vi "Pick Up and Go.vi"(0 "Feet":dbl=10.0 format="%#_13g") -> ()   [LabVIEW 2014]
panel:
  in  "Time":i32
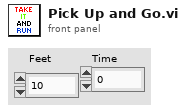
[diagram p1: front panel]
types:
  T1 = enum16{"Move Forward", "Move Backward", "Strafe Right", "Strafe Left"}
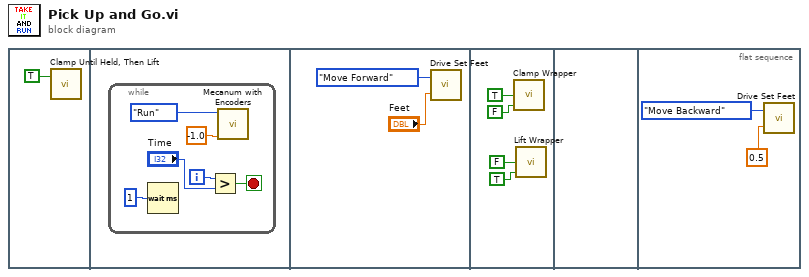
[diagram p0: block diagram]
diagram:
  n1 = flat-sequence {
    frame #0 {
      n2 = call "Clamp Until Held, Then Lift.vi"("Clamp + Lift"=TRUE) -> ()  [unwired: 2 in]
    }
    frame #1 {
      n3 = while {
        i -> [w4]
        stop <- w6 stop-if-true
        n4 = Wait (ms)(milliseconds to wait=u32 1) -> ()  [unwired: 1 out]
        n5 = Greater?(x=w4, y="Time") -> (0:w6:bool)
        n6 = call "Mecanum with Encoders.vi"("Turn"=-1.0, "Mode"=enum8{"Start", "Run", "Finish"}."Run") -> ()  [unwired: 8 in, 1 out]
      }
    }
    frame #2 {
      n7 = call "Drive Set Feet.vi"("Feet"="Feet", "Direction"=T1."Move Forward") -> ()  [unwired: 1 out]
    }
    frame #3 {
      n8 = call "Clamp Wrapper.vi"("In"=FALSE, "Out"=TRUE) -> ()  [unwired: 1 in]
      n9 = call "Lift Wrapper.vi"("Down"=TRUE, "Up"=FALSE) -> ()  [unwired: 1 in]
    }
    frame #4 {
    }
    frame #5 {
      n10 = call "Drive Set Feet.vi"("Feet"=0.5 ("Feet 2"), "Direction"=T1."Move Backward") -> ()  [unwired: 1 out]
    }
  }
